vi "ODD EVEN.vi"() -> ()   [LabVIEW 2018]
panel:
  out "Boolean 2":bool
  out "Boolean":bool
  in  "Numeric":dbl
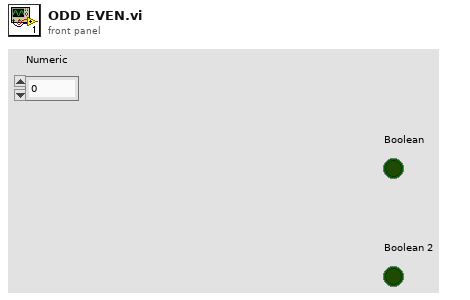
[diagram p1: front panel]
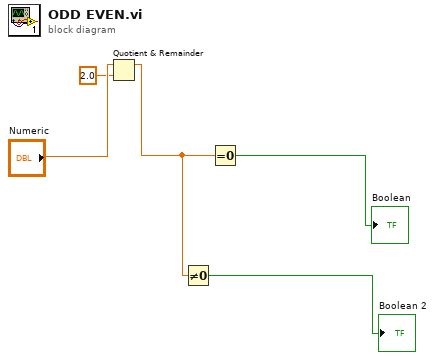
[diagram p0: block diagram]
diagram:
  n1 = Quotient & Remainder(x="Numeric", y=2.0) -> (x-y*floor(x/y)=w1:dbl)  [unwired: 1 out]
  n2 = Not Equal To 0?(x=w1) -> (x != 0?=→"Boolean 2":bool)
  n3 = Equal To 0?(x=w1) -> (x = 0?=→"Boolean":bool)
